vi "Wrap Execution Ref.vi"(8 "error in (no error)":errorcluster, 10 "Execution Ref":refnum<k7>, 11 "Engine in":refnum<class "Engine.lvclass">) -> (0 "error out":errorcluster, 2 "Execution":refnum<class "Execution.lvclass">, 3 "Engine out":refnum<class "Engine.lvclass">)   [LabVIEW 2020, in "TSnax.lvlib" / "Engine.lvclass"]
uses:
  Engine.lvclass
  Execution/Execution.lvclass
  Engine.lvclass/Engine.ctl
  <vilib>/Utility/miscctls.llb/LVMapReplaceAction.ctl
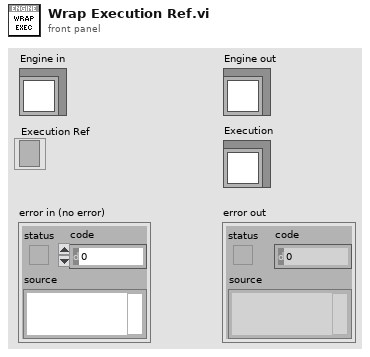
[diagram p1: front panel]
types:
  T1 = typedef "LVMapReplaceAction.ctl" = enum32{"Modify Entry only if found", "Add or Modify Entry", "Delete Entry"}
  T2 = typedef "TSnax.lvlib/Engine.lvclass/Ref Data.ctl" = cluster{"Station Globals":refnum<class "PropertyObject.lvclass">, "Station Model":refnum<class "SequenceFile.lvclass">, "Trace Delay":u32, "Execution Map":map{i32, refnum<class "Execution.lvclass">}}
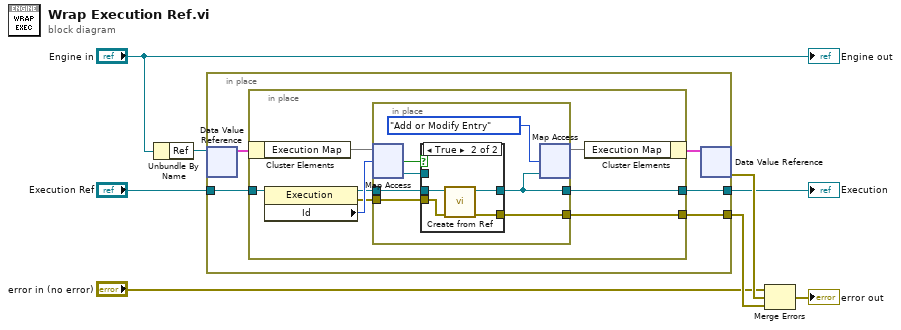
[diagram p0: block diagram]
diagram:
  n1 = Unbundle By Name("Engine in") -> ("Ref"=w7:refnum<data-value>)
  n2 = in-place {
    in-place-border: "Execution Ref" -> [w11]
    in-place-border: [w10] -> w4
    in-place-border: [w9] -> w3
    n3 = in-place-dvr #1(w7) -> (w13:T2)  [unwired: 1 out]
    n4 = in-place {
      in-place-border: w11 -> [w19]
      in-place-border: [w16] -> w10
      in-place-border: [w14] -> w9
      n5 = in-place-cluster #2(w13) -> ("Execution Map"=w21:map{i32, refnum<class "Execution.lvclass">})
      n6 = property class="Execution"(reference=w19) -> (reference out=w17:refnum<k7>, error out=w15:errorcluster, "Id"=w18:i32)  [unwired: 1 in]
      n7 = in-place {
        in-place-border: w17 -> [w26]
        in-place-border: [w24] -> w16
        in-place-border: w15 -> [w23]
        in-place-border: [w22] -> w14
        n8 = in-place-map #3(w21, w18) -> (w27:refnum<class "Execution.lvclass">, w28:bool)  [unwired: 1 in]
        n9 = case shown="True" w28 {
          tunnel: w27 -> [w30 _]
          tunnel: w26 -> [_ w34]
          tunnel: [w30 w33] -> w24
          tunnel: w23 -> [w29 w32]
          tunnel: [w29 w31] -> w22
          frame False {
          }
          frame True {
            n10 = call "Create from Ref.vi"("error in (no error)"=w32, "Execution Ref"=w34) -> ("error out"=w31:errorcluster, "Execution out"=w33:refnum<class "Execution.lvclass">)  [unwired: 8 in]
          }
        }
        n11 = in-place-map #3(w24, LVMapReplaceAction."Add or Modify Entry" ("action")) -> (w20:map{i32, refnum<class "Execution.lvclass">})  [unwired: 2 out]
      }
      n12 = in-place-cluster #2("Execution Map"=w20) -> (w12:T2)
    }
    n13 = in-place-dvr #1(w12) -> (w8:errorcluster)  [unwired: 1 out]
  }
  "Execution" <- w4
  n14 = Merge Errors("error in (no error)", w8, w3) -> (→"error out":errorcluster)
  "Engine out" <- "Engine in"
